vi "Receive Chat Message.vi"(8 "error in (no error)":errorcluster, 9 "Message":string, 10 "Sender":string, 11 "Simple Chat in":refnum<class "Simple Chat.lvclass">) -> (0 "error out":errorcluster, 3 "Simple Chat out":refnum<class "Simple Chat.lvclass">)   [LabVIEW 2020, in "Simple Chat.lvlib" / "Simple Chat.lvclass"]
uses:
  Simple Chat.lvclass
  Simple Chat.lvclass/Simple Chat.ctl
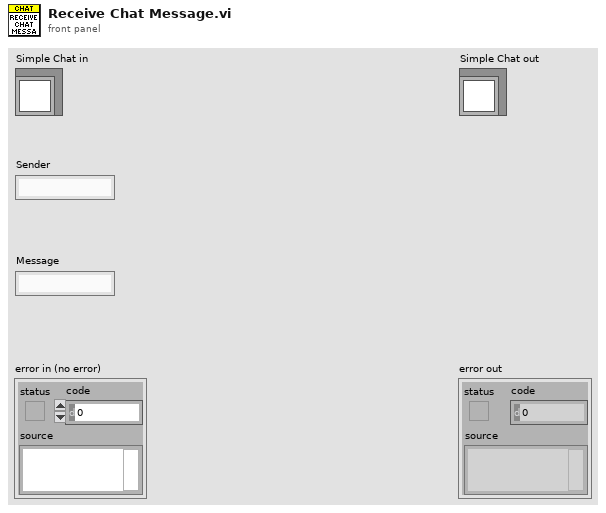
[diagram p1: front panel]
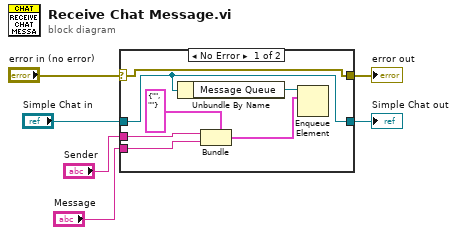
[diagram p0: block diagram]
diagram:
  n1 = case shown="No Error" "error in (no error)" {
    selector: "error in (no error)" -> [w13 w15]
    tunnel: [w13 w15] -> w5
    tunnel: [w12 w14] -> w3
    tunnel: "Simple Chat in" -> [w12 w14]
    tunnel: "Sender" -> [w8 _]
    tunnel: "Message" -> [w7 _]
    frame No Error {
      n2 = Unbundle By Name(w12) -> ("Message Queue"=w11:refnum<queue>)
      n3 = Bundle(cluster=cluster{"Sender":string, "Message":string} {"Sender"="", "Message"=""} ("element"), "Sender"=w8, "Message"=w7) -> (w9:cluster{"Sender":string, "Message":string})
      n4 = Enqueue Element(queue=w11, element=w9) -> ()  [unwired: 2 in, 3 out]
    }
    frame Error {
    }
  }
  "error out" <- w5
  "Simple Chat out" <- w3
